vi "example_scan_continuous.vi"() -> ()   [LabVIEW 2021, in "libad4.lvlib"]
uses:
  <userlib>/libad4/libad4.lvlib
  <userlib>/libad4/controls/init scan cha desc.ctl
  <userlib>/libad4/controls/ad scan desc.ctl
panel:
  out "Digital Graph":waveform(sgl)(graph)
  out "Analog Graph":waveform(sgl)(graph)
  out "sd out":T1
  in  "DAQ ID":string="usbbase"
  in  "ad_scan_desc":T1={"sample_rate"=0.001, "clock_rate"=0.0, "prehist"=0, "posthist"=1000, "ticks_per_run"=100, "bytes_per_run"=0, "samples_per_run"=0, "flags"=0, "sd_res[0]"=0, "sd_res[1]"=0, "sd_res[2]"=0, "sd_res[3]"=0, "sd_res[4]"=0, "sd_res[5]"=0, "sd_res[6]"=0, "sd_res[7]"=0, "sd_res[8]"=0, "sd_res[9]"=0, "sd_res[10]"=0, "sd_res[11]"=0}
  in  "cha_desc_vector":T2[](array[typedef])=[{"Channel Type"=enum."AD_CHA_TYPE_ANALOG_IN", "Channel No."=1, "range"=0, "Store type"=[enum."AD_STORE_DISCRETE"], "ratio"=1, "zero"=0, "trg_mode"=enum."AD_TRG_NONE", "trg_par[0]"=0, "trg_par[1]"=0}, {"Channel Type"=enum."AD_CHA_TYPE_DIGITAL_IO", "Channel No."=2, "range"=0, "Store type"=[enum."AD_STORE_DISCRETE"], "ratio"=2, "zero"=0, "trg_mode"=enum."AD_TRG_NONE", "trg_par[0]"=0, "trg_par[1]"=0}]
  # "Scan Analog channel 1 and Digital channel 1"
  # "Input parameters"
  # "Output data"
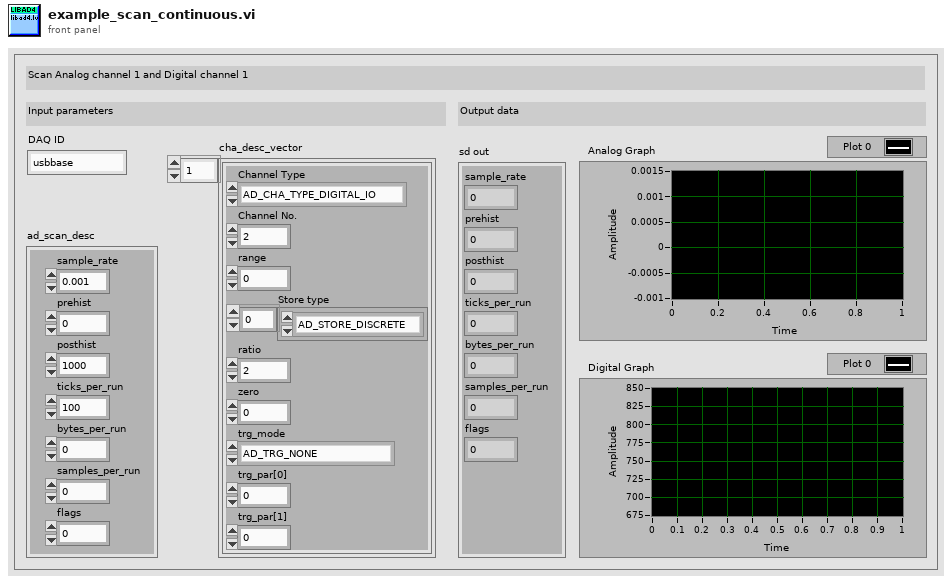
[diagram p1: front panel]
types:
  T1 = typedef "libad4.lvlib/ad scan desc.ctl" = cluster{"sample_rate":dbl, "clock_rate":dbl, "prehist":u64, "posthist":u64, "ticks_per_run":u32, "bytes_per_run":u32, "samples_per_run":u32, "flags":u32, "sd_res[0]":u32, "sd_res[1]":u32, "sd_res[2]":u32, "sd_res[3]":u32, "sd_res[4]":u32, "sd_res[5]":u32, "sd_res[6]":u32, "sd_res[7]":u32, "sd_res[8]":u32, "sd_res[9]":u32, "sd_res[10]":u32, "sd_res[11]":u32}
  T2 = typedef "libad4.lvlib/init scan cha desc.ctl" = cluster{"Channel Type":enum16{"AD_CHA_TYPE_ANALOG_IN", "AD_CHA_TYPE_ANALOG_OUT", "AD_CHA_TYPE_DIGITAL_IO"}, "Channel No.":i32, "range":i32, "Store type":enum16{"AD_STORE_DISCRETE", "AD_STORE_AVERAGE", "AD_STORE_MIN", "AD_STORE_MAX", "AD_STORE_RMS"}[], "ratio":i32, "zero":u32, "trg_mode":enum16{"AD_TRG_NONE", "AD_TRG_POSITIVE", "AD_TRG_NEGATIVE", "AD_TRG_INSIDE", "AD_TRG_OUTSIDE", "AD_TRG_NEVER"}, "trg_par[0]":u32, "trg_par[1]":u32}
  T3 = typedef "libad4.lvlib/ad scan cha desc.ctl" = cluster{"cha":i32, "range":i32, "store":i32, "ratio":i32, "zero":u32, "trg_mode":u8, "alarm_mode":u8, "sc_res1[0]":u8, "sc_res1[1]":u8, "trg_par[0]":u32, "trg_par[1]":u32, "samples_per_run":i32, "alarm_par[0]":u32, "alarm_par[1]":u32, "sc_res2[0]":u32, "sc_res2[1]":u32, "sc_res2[2]":u32, "sc_res2[3]":u32, "sc_res2[4]":u32}
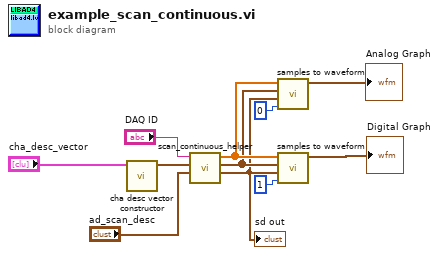
[diagram p0: block diagram]
diagram:
  n1 = call <userlib>:"cha desc vector constructor.vi"("init_cha_desc_vec"="cha_desc_vector") -> ("ad_scan_cha_desc_vec"=w10:T3[])  [unwired: 10 in]
  n2 = call <userlib>:"scan_continuous_helper.vi"("scan_desc"="ad_scan_desc", "chav"=w10, "DAQ ID"="DAQ ID") -> ("scan_desc out"=w1:T1, "chav out"=w2:T3[], "data"=w3:sgl[])  [unwired: 5 in, 1 out]
  "sd out" <- w1
  n3 = call <userlib>:"samples to waveform.vi"("Channel ID (row)"=0, "ad_scan_desc"=w1, "chav in"=w2, "buffer in"=w3) -> ("Waveform"=→"Analog Graph":waveform(sgl))  [unwired: 7 in]
  n4 = call <userlib>:"samples to waveform.vi"("Channel ID (row)"=1, "ad_scan_desc"=w1, "chav in"=w2, "buffer in"=w3) -> ("Waveform"=→"Digital Graph":waveform(sgl))  [unwired: 7 in]
